vi "MissingFileFolder.vi"() -> ()   [LabVIEW 2016]
panel:
  out "Missing Folder":path[](array[path])
  out "Missing Files":path[](array[path])
  in  "Folder Path 2":path
  in  "Folder Path":path
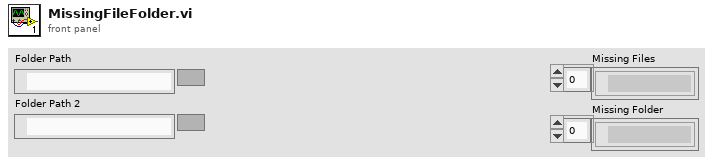
[diagram p1: front panel]
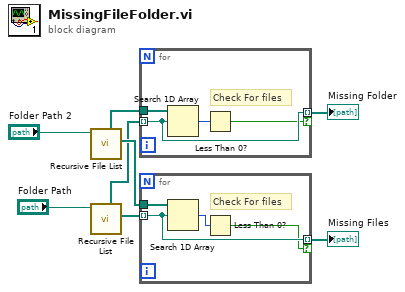
[diagram p0: block diagram]
diagram:
  n1 = call <vilib>:"Recursive File List.vi"("Folder Path"="Folder Path 2") -> ("All Files in Dir"=w5:path[], "All Folders"=w2:path[])  [unwired: 6 in, 3 out]
  n2 = call <vilib>:"Recursive File List.vi"("Folder Path"="Folder Path") -> ("All Files in Dir"=w6:path[], "All Folders"=w3:path[])  [unwired: 6 in, 3 out]
  n3 = for {
    tunnel: w3 -> [w10] mode=indexing
    tunnel: w2 -> [w12]
    tunnel: [w10] -> w1 mode=indexing if=w9
    # "Check For files"
    n4 = Search 1D Array(1D array=w12, element=w10) -> (index of element=w11:i32)  [unwired: 1 in]
    n5 = Less Than 0?(x=w11) -> (x < 0?=w9:bool)
  }
  "Missing Folder" <- w1
  n6 = for {
    tunnel: w6 -> [w14] mode=indexing
    tunnel: w5 -> [w16]
    tunnel: [w14] -> w4 mode=indexing if=w13
    # "Check For files"
    n7 = Search 1D Array(1D array=w16, element=w14) -> (index of element=w15:i32)  [unwired: 1 in]
    n8 = Less Than 0?(x=w15) -> (x < 0?=w13:bool)
  }
  "Missing Files" <- w4
